vi "PerformMeasure.vi"(2 "Command":string="ft\n", 3 "error in":errorcluster, 4 "Serial Communication Port:":refnum<visa-resource-name>="COM1") -> (0 "Response":string, 1 "error out":errorcluster)   [LabVIEW 2019]
uses:
  SerialConfig.ctl
  ParityInfo.ctl
  FlowControlInfo.ctl
  <vilib>/Instr/_visa.llb/VISA Configure Serial Port (Instr).vi
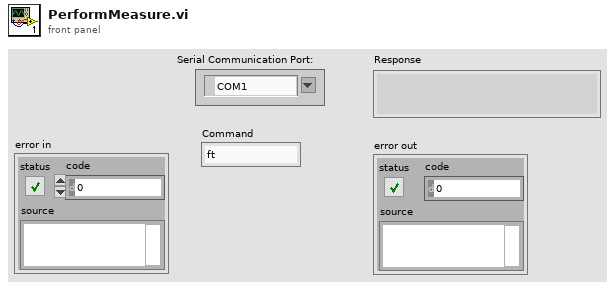
[diagram p1: front panel]
types:
  T1 = typedef "SerialConfig.ctl" = cluster{"Baud":u32, "Data Bits":u16, "Stop bits":u16, "Parity":T2, "flow control":T3}
  T2 = typedef "ParityInfo.ctl" = enum16{"None", "Odd", "Even", "Mark", "Space"}
  T3 = typedef "FlowControlInfo.ctl" = u16
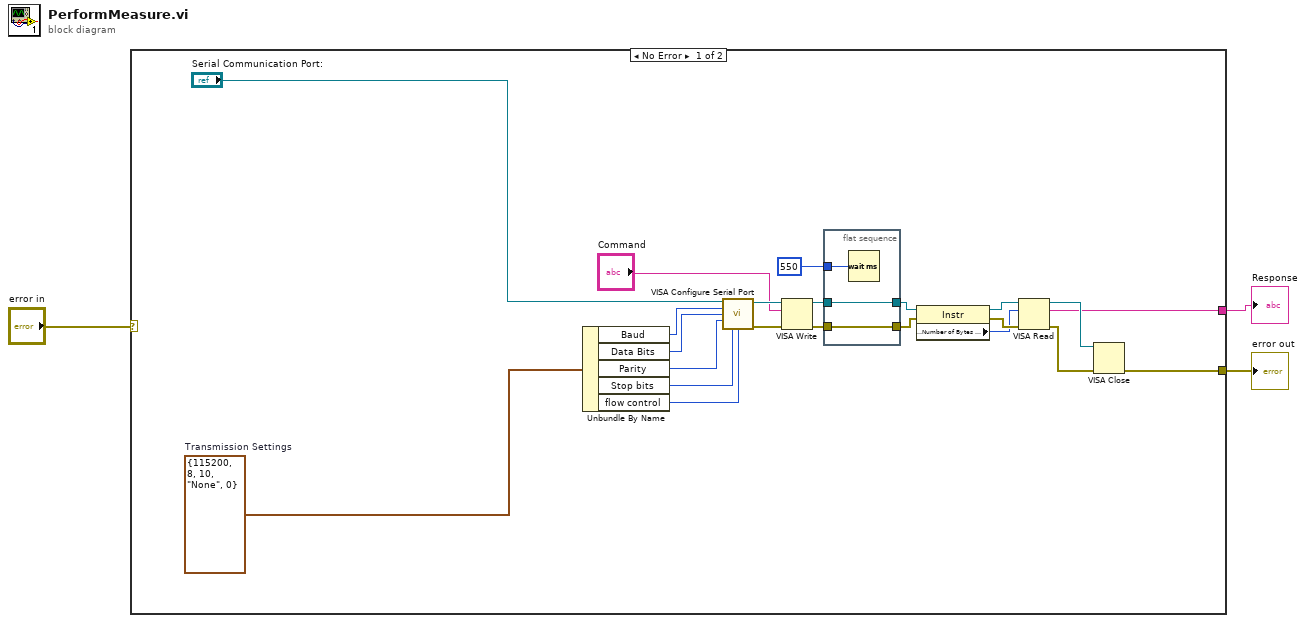
[diagram p0: block diagram]
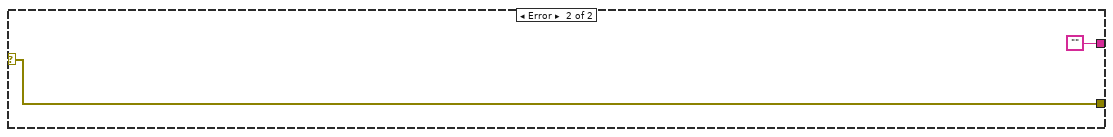
[diagram p2: hidden frame]
diagram:
  n1 = case shown="No Error" "error in" {
    selector: "error in" -> [_ w30]
    tunnel: [w5 w30] -> w3
    tunnel: [w4 ""] -> w2
    frame No Error {
      w8 = T1 {"Baud"=115200, "Data Bits"=8, "Stop bits"=10, "Parity"=enum."None", "flow control"=0}  # Transmission Settings
      n2 = Unbundle By Name(w8) -> ("Baud"=w11:u32, "Data Bits"=w10:u16, "Parity"=w7:T2, "Stop bits"=w9:u16, "flow control"=w13:T3)
      n3 = call-poly "VISA Configure Serial Port"("VISA resource name"="Serial Communication Port:", "baud rate (9600)"=w11, "data bits (8)"=w10, "parity (0:none)"=w7, "stop bits (10: 1 bit)"=w9, "flow control (0:none)"=w13) -> ("VISA resource name out"=w23:refnum<visa-resource-name>, "error out"=w24:errorcluster)  [unwired: 3 in, 5 out]
      n4 = VISA Write(VISA resource name=w23, write buffer="Command", error in (no error)=w24) -> (VISA resource name out=w18:refnum<visa-resource-name>, error out=w20:errorcluster)  [unwired: 1 out]
      n5 = flat-sequence {
        tunnel: w20 -> [w28]
        tunnel: [w28] -> w19
        tunnel: w18 -> [w27]
        tunnel: [w27] -> w17
        tunnel: 550 -> [w26]
        frame #0 {
          n6 = Wait (ms)(milliseconds to wait=w26) -> ()  [unwired: 1 out]
        }
      }
      n7 = property class="Instr"(reference=w17, error in=w19) -> (reference out=w16:refnum<visa-resource-name>, error out=w15:errorcluster, "Serial Settings:Number of Bytes at Serial Port"=w14:u32)
      n8 = VISA Read(VISA resource name=w16, byte count=w14, error in (no error)=w15) -> (VISA resource name out=w21:refnum<visa-resource-name>, read buffer=w4:string, error out=w22:errorcluster)  [unwired: 1 out]
      n9 = VISA Close(VISA resource name=w21, error in (no error)=w22) -> (error out=w5:errorcluster)
    }
    frame Error {
    }
  }
  "error out" <- w3
  "Response" <- w2
